vi "AutoDriveForward.vi"(8 "error in (no error)":errorcluster) -> (0 "error out":errorcluster)   [LabVIEW 2013]
uses:
  <vilib>/Rock Robotics/WPI/RobotDrive/WPI_RobotDriveGetSetRefNum.vi
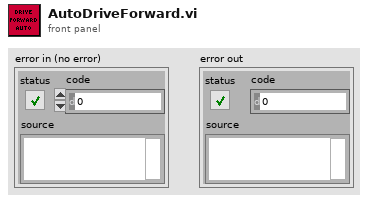
[diagram p1: front panel]
types:
  T1 = typedef "WPI_RobotDriveDevRef.ctl" = cluster{"DevStatus":errorcluster, "Motors[]":T2[], "Square Inputs":bool, "Max Output":dbl, "Isochronous":bool}
  T2 = typedef "WPI_MotorControlDeviceRef.ctl" = cluster{"DeviceStatus":errorcluster, "Type":enum16{"PWM", "CAN"}, "PWM":cluster{"Digital Module":T3, "PWM Channel":T4, "DeadBand":T5}, "CAN":cluster{"Device Number":u8, "Control Mode":T6, "Semaphore":T7, "Max Vout":dbl}, "Invert":bool, "TransformRef":T8, "InvTransformRef":T8}
  T3 = typedef "FPGA_TypedefDigitalModule.ctl" = enum16{"Digital Module 1", "Digital Module 2"}
  T4 = typedef "FPGA_DIOPWMChannel.ctl" = enum8{"PWM 1", "PWM 2", "PWM 3", "PWM 4", "PWM 5", "PWM 6", "PWM 7", "PWM 8", "PWM 9", "PWM 10", "Invalid"}
  T5 = typedef "WPI_PWMDeadband.ctl" = cluster{"Name":string, "maxPositivePwm":i32, "minPositivePwm":i32, "centerPwm":i32, "maxNegativePwm":i32, "minNegativePwm":i32, "angularRange":u16}
  T6 = typedef "WPI_CANJaguar_ControlMode.ctl" = enum8{"Percent VBus", "Current", "Speed", "Position", "Voltage"}
  T7 = typedef "Semaphore RefNum" = refnum<k1>
  T8 = typedef "WPI_PWMTransform_ConPane.ctl" = refnum<vi>
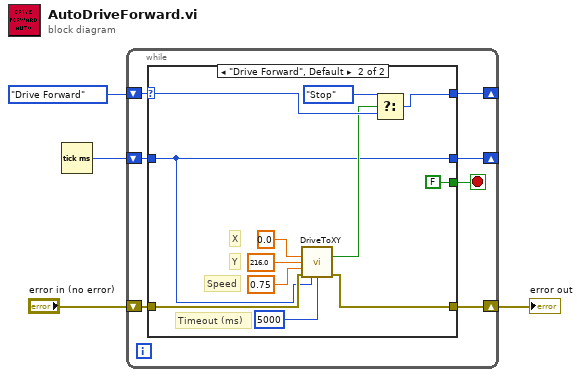
[diagram p0: block diagram]
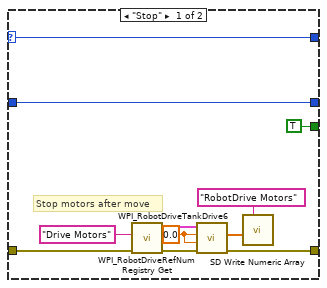
[diagram p2: hidden frame]
diagram:
  n1 = Tick Count (ms)() -> (millisecond timer value=w4:u32)
  n2 = while {
    shift-right: [w8] -> _
    shift-left: enum16{"Drive Forward", "Stop"}."Drive Forward" -> [w11]
    shift-right: [w9] -> w3
    shift-left: "error in (no error)" -> [w10]
    shift-right: [w6] -> _
    shift-left: w4 -> [w7]
    stop <- w5 stop-if-true
    n3 = case shown="\"Drive Forward\", Default" w11 {
      selector: w11 -> [w14 w28]
      tunnel: w10 -> [w19 w31]
      tunnel: [w17 w30] -> w9
      tunnel: [w14 w27] -> w8
      tunnel: w7 -> [w15 w23]
      tunnel: [w15 w23] -> w6
      tunnel: [TRUE FALSE] -> w5
      frame "Stop" {
        w20 = 0.0 ("Left axis value")
        # "Stop motors after move"
        n4 = call <vilib>:"WPI_RobotDriveRefNum Registry Get.vi"("error in (no error)"=w19, "refnum name"="Drive Motors") -> ("error out"=w18:errorcluster, "RobotDriveDevRef"=w22:T1)  [unwired: 8 out]
        n5 = call "WPI_RobotDriveTankDrive6.vi"("error in (no error)"=w18, "Right axis value"=w20, "Left axis value"=w20, "RobotDriveDevRef"=w22) -> ("error out"=w17:errorcluster, "Motor Values"=w12:dbl[])  [unwired: 5 in, 1 out]
        n6 = call <vilib>:"SD Write Numeric Array.vi"("Numeric Array"=w12, "Name"="RobotDrive Motors") -> ()  [unwired: 8 in, 2 out]
      }
      frame "Drive Forward", Default {
        # "Timeout (ms)"
        # "Speed"
        # "Y"
        # "X"
        n7 = call "DriveToXY.vi"("X Target"=0.0, "Y Target"=216.0, "Speed"=0.75, "error in"=w31, "Start time"=w23, "Timeout (ms)"=u32 5000 ("y")) -> ("At Target"=w26:bool, "error out"=w30:errorcluster)  [unwired: 6 in, 2 out]
        n8 = Select(t=enum16{"Drive Forward", "Stop"}."Stop", s=w26, f=w28) -> (s? t:f=w27:enum16{"Drive Forward", "Stop"})
      }
    }
  }
  "error out" <- w3
